vi "Switch On Button Press.vi"(1 "Button":bool) -> (0 "Output":bool)   [LabVIEW 2018]
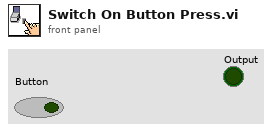
[diagram p1: front panel]
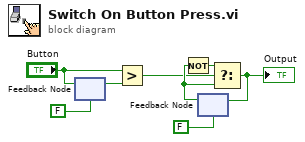
[diagram p0: block diagram]
diagram:
  n1 = feedback #1(FALSE ("Button")) -> (w3:bool)
  n2 = feedback-in #1("Button") -> ()
  n3 = Greater?(x="Button", y=w3) -> (0:w5:bool)
  n4 = feedback #2(FALSE) -> (w7:bool)
  n5 = Not(x=w7) -> (.not. x?=w6:bool)
  n6 = Select(t=w6, s=w5, f=w7) -> (s? t:f=w8:bool)
  "Output" <- w8
  n7 = feedback-in #2(w8) -> ()
